vi "ELVIS III v1.1 Register AI IRQ.vi"(3 "Hysteresis (0.02)":dbl=0.02 format="%#_13g", 4 "Callback VI Reference":T2, 5 "Allow Overwrite Operation? (F)":bool, 6 "Threshold":dbl=2.5, 7 "IRQ Number":u8, 8 "error in (no error)":errorcluster, 9 "Analog Interrupt Type":T3, 10 "Channel Name":string, 11 "Resource name":T1 caption="RIO Device") -> (0 "error out":errorcluster)   [LabVIEW 2021]
uses:
  <vilib>/myRIO/Common/Instrument Driver Framework/myRIO v1.0/IRQ/typedefs/AI IRQ Type.ctl
  <vilib>/myRIO/Common/Instrument Driver Framework/myRIO v1.0/IRQ/typedefs/Callback VI Ref.ctl
  <vilib>/userDefined/High Color/nirio_resource_hc.ctl
  <vilib>/myRIO/Common/Instrument Driver Framework/myRIO v1.0/IRQ/typedefs/IRQ Type.ctl
  <vilib>/myRIO/Common/Instrument Driver Framework/myRIO v1.0/IRQ/typedefs/IO IRQ Channels Enum.ctl
  <vilib>/myRIO/Common/Instrument Driver Framework/ELVIS III v1.0/IRQ/typedefs/ELVIS III v1.0 AI IRQ Channels Enum.ctl
  <vilib>/Utility/VariantDataType/GetNumericInfo.vi
  <vilib>/Utility/error.llb/Error Cluster From Error Code.vi
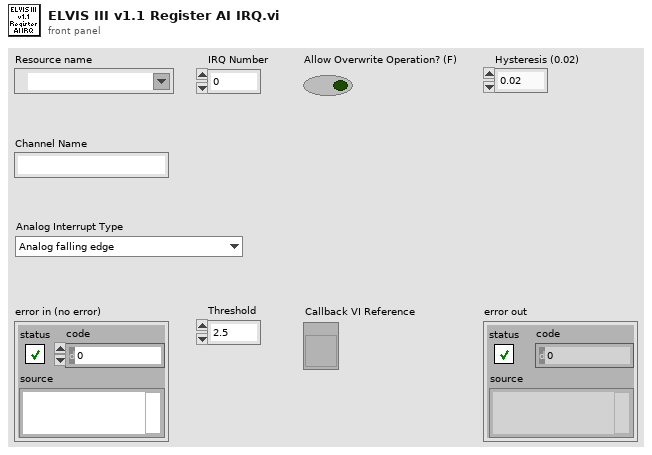
[diagram p1: front panel]
types:
  T1 = typedef "nirio_resource_hc.ctl" = tag
  T2 = typedef "Callback VI Ref.ctl" = refnum<vi>
  T3 = typedef "AI IRQ Type.ctl" = enum16{"Analog falling edge", "Analog rising edge"}
  T4 = typedef "IRQ Type.ctl" = enum16{"Timer", "Analog falling edge", "Analog rising edge", "Digital falling edge", "Digital rising edge", "Digital edge"}
  T5 = typedef "IO IRQ Channels Enum.ctl" = enum16{"Not Connected", "A/AI0 (Interrupt)", "A/AI1 (Interrupt)", "A/DIO0 (Interrupt)", "A/DIO1 (Interrupt)", "A/DIO2 (Interrupt)", "A/DIO3 (Interrupt)", "Button0 (Interrupt)", "B/AI0 (Interrupt)", "B/AI1 (Interrupt)", "B/DIO0 (Interrupt)", "B/DIO1 (Interrupt)", "B/DIO2 (Interrupt)", "B/DIO3 (Interrupt)"}
  T6 = typedef "ELVIS III v1.0 AI IRQ Channels Enum.ctl" = enum16{"Not Connected", "A/AI0 (Interrupt)", "A/AI1 (Interrupt)"}
  T7 = typedef "Generic FPGA Reference.ctl" = refnum<k20>
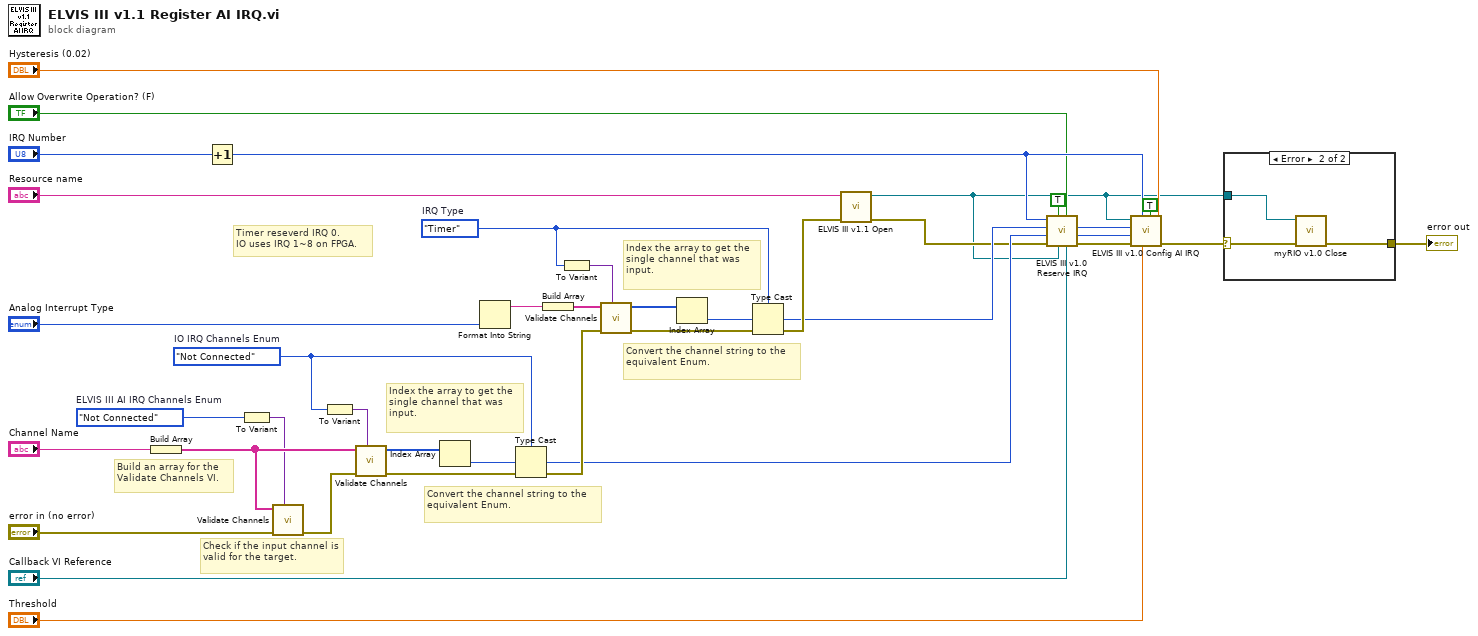
[diagram p0: block diagram]
diagram:
  w22 = IRQ_Type."Timer"  # IRQ Type
  w26 = IO_IRQ_Channels_Enum."Not Connected"  # IO IRQ Channels Enum
  w29 = ELVIS_III_v1.0_AI_IRQ_Channels_Enum."Not Connected"  # ELVIS III AI IRQ Channels Enum
  # "Timer reseverd IRQ 0.\nIO uses IRQ 1~8 on FPGA."
  # "Index the array to get the single channel that was input."
  # "Convert the channel string to the equivalent Enum."
  # "Index the array to get the single channel that was input."
  # "Build an array for the Validate Channels VI."
  # "Convert the channel string to the equivalent Enum."
  # "Check if the input channel is valid for the target."
  n1 = Build Array("Channel Name") -> (w33:string[])
  n2 = Increment(x="IRQ Number") -> (x+1=w7:u8)
  n3 = To Variant(anything=w29) -> (Variant=w28:variant)
  n4 = call <vilib>:"Validate Channels.vi"("Channels Enum Variant"=w28, "error in (no error)"="error in (no error)", "Channel Names"=w33) -> ("error out"=w32:errorcluster)  [unwired: 7 in, 1 out]
  n5 = To Variant(anything=w26) -> (Variant=w27:variant)
  n6 = call <vilib>:"Validate Channels.vi"("Channels Enum Variant"=w27, "error in (no error)"=w32, "Channel Names"=w33) -> ("error out"=w20:errorcluster, "Index Array"=w34:u16[])  [unwired: 7 in]
  n7 = Index Array(array=w34) -> (element=w35:u16)  [unwired: 1 in]
  n8 = Format Into String("Analog Interrupt Type") -> (resulting string=w9:string)  [unwired: 3 in, 1 out]
  n9 = Type Cast(type=w26, x=w35) -> (*(type *) &x=w4:T5)
  n10 = Build Array(w9) -> (w21:string[])
  n11 = To Variant(anything=w22) -> (Variant=w25:variant)
  n12 = call <vilib>:"Validate Channels.vi"("Channels Enum Variant"=w25, "error in (no error)"=w20, "Channel Names"=w21) -> ("error out"=w12:errorcluster, "Index Array"=w24:u16[])  [unwired: 7 in]
  n13 = Index Array(array=w24) -> (element=w23:u16)  [unwired: 1 in]
  n14 = Type Cast(type=w22, x=w23) -> (*(type *) &x=w5:T4)
  n15 = call <vilib>:"ELVIS III v1.1 Open.vi"("error in (no error)"=w12, "Resource name"="Resource name") -> ("error out"=w2:errorcluster, "myRIO FPGA Ref Out"=w1:T7)  [unwired: 8 in]
  n16 = call <vilib>:"ELVIS III v1.0 Reserve IRQ.vi"("Callback VI Ref"="Callback VI Reference", "Allow Overwrite? (F)"="Allow Overwrite Operation? (F)", "myRIO FPGA Ref In"=w1, "Is Reserve?"=TRUE, "error in (no error)"=w2, "IO IRQ Channels Enum"=w4, "IRQ Type"=w5, "IRQ Number"=w7) -> ("error out"=w18:errorcluster)  [unwired: 2 in, 1 out]
  n17 = call <vilib>:"ELVIS III v1.0 Config AI IRQ.vi"("Hysteresis"="Hysteresis (0.02)", "Enable IRQ?"=TRUE, "Threshold"="Threshold", "IRQ Number"=w7, "error in (no error)"=w18, "IO IRQ Channels Enum"=w4, "IRQ Type"=w5, "myRIO FPGA Ref In"=w1) -> ("error out"=w15:errorcluster)  [unwired: 3 in]
  n18 = case shown="Error" w15 {
    selector: w15 -> [w36 w39]
    tunnel: w1 -> [_ w37]
    tunnel: [w36 w38] -> w14
    frame No Error {
    }
    frame Error {
      n19 = call <vilib>:"myRIO v1.0 Close.vi"("error in (no error)"=w39, "myRIO FPGA Ref In"=w37) -> ("error out"=w38:errorcluster)  [unwired: 9 in]
    }
  }
  "error out" <- w14
